vi "kalman pv measurement step fixed gain.vi"(8 "v gain":fxp<+,16,0> format="%.16g", 9 "x gain":fxp<+,16,0> format="%.16g", 10 "position measurement":i16, 11 "Kalman PV state":T1) -> (3 "kalman pv state out":T1)   [LabVIEW 2010]
uses:
  kalman pv state.ctl
  <vilib>/rvi/FXPMathLib/FxpSub/XNode/nifxpmath_Sub.xnode
  <vilib>/rvi/FXPMathLib/FxpSub/subVIs/nifxpmath_Sub_SimConfig.ctl
  <vilib>/fxp/LVFixedPointQuantizationPolicyTypeDef.ctl
  <vilib>/fxp/LVFixedPointOverflowPolicyTypeDef.ctl
  <vilib>/rvi/FXPMathLib/FxpMul/XNode/nifxpmath_Multiplier.xnode
  <vilib>/rvi/FXPMathLib/FxpMul/subVIs/nifxpmath_Mul_SimConfig.ctl
  <vilib>/rvi/FXPMathLib/FxpAdd/XNode/nifxpmath_Add.xnode
  <vilib>/rvi/FXPMathLib/FxpAdd/subVIs/nifxpmath_Add_SimConfig.ctl
  <vilib>/rvi/FXPMathLib/FxpSub/simVIs/DllFxpSubTemp_sub.vi
  <vilib>/rvi/FXPMathLib/FxpMul/simVIs/DllFxpMulTemp_sub.vi
  <vilib>/rvi/FXPMathLib/FxpAdd/simVIs/DllFxpAddTemp_sub.vi
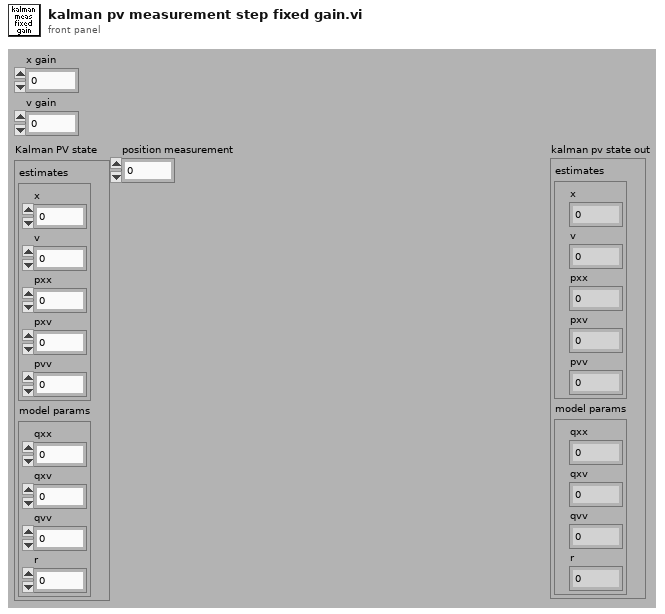
[diagram p1: front panel]
types:
  T1 = typedef "kalman pv state.ctl" = cluster{"estimates":cluster{"x":fxp<+/-,18,16>, "v":fxp<+/-,18,16>, "pxx":u16, "pxv":u16, "pvv":u16}, "model params":cluster{"qxx":u16, "qxv":u16, "qvv":u16, "r":u16}}
  T2 = cluster{"x":fxp<+/-,18,16>, "v":fxp<+/-,18,16>, "pxx":u16, "pxv":u16, "pvv":u16}
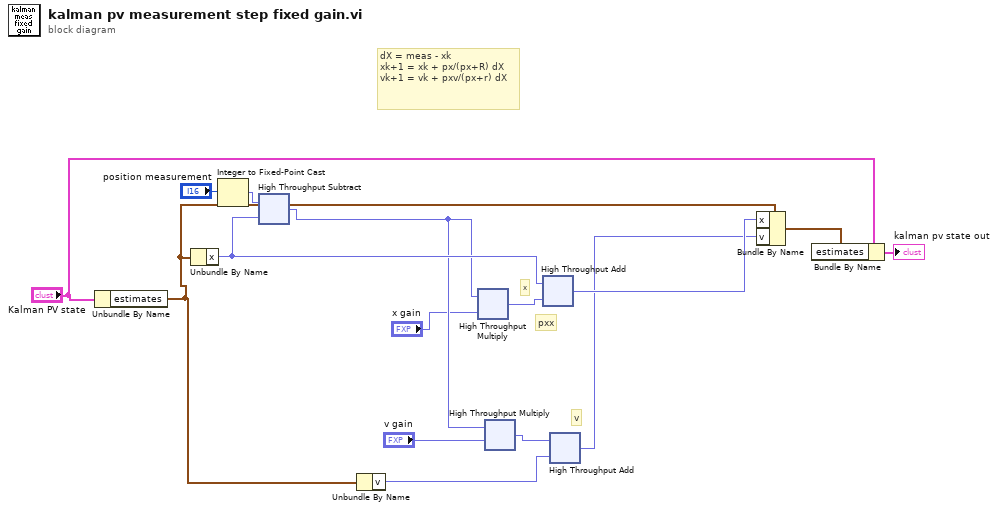
[diagram p0: block diagram]
diagram:
  # "dX = meas - xk\nxk+1 = xk + px/(px+R) dX\nvk+1 = vk + pxv/(px+r) dX"
  # "v"
  # "pxx"
  # "x"
  n1 = Unbundle By Name("Kalman PV state") -> ("estimates"=w14:T2)
  n2 = Unbundle By Name(w14) -> ("x"=w6:fxp<+/-,18,16>)
  n3 = Integer to Fixed-Point Cast(integer="position measurement") -> (fixed-point=w4:fxp<+/-,16,16>)  [unwired: 1 in]
  n4 = xnode "High Throughput Subtract"("x"=w4, "y"=w6) -> ("x-y"=w3:fxp<+/-,18,16>)
  n5 = Unbundle By Name(w14) -> ("v"=w8:fxp<+/-,18,16>)
  n6 = xnode "High Throughput Multiply"("x"=w3, "y"="x gain") -> ("x*y"=w15:fxp<+/-,18,16>)
  n7 = xnode "High Throughput Multiply"("x"=w3, "y"="v gain") -> ("x*y"=w9:fxp<+/-,18,16>)
  n8 = xnode "High Throughput Add"("x"=w6, "y"=w15) -> ("x+y"=w13:fxp<+/-,18,16>)
  n9 = xnode "High Throughput Add"("x"=w9, "y"=w8) -> ("x+y"=w7:fxp<+/-,18,16>)
  n10 = Bundle By Name(cluster=w14, "x"=w13, "v"=w7) -> (w12:T2)
  n11 = Bundle By Name(cluster="Kalman PV state", "estimates"=w12) -> (→"kalman pv state out":T1)
